vi "tables.vi"() -> ()   [LabVIEW 2018]
panel:
  out "Array":i32[][](array[numeric])
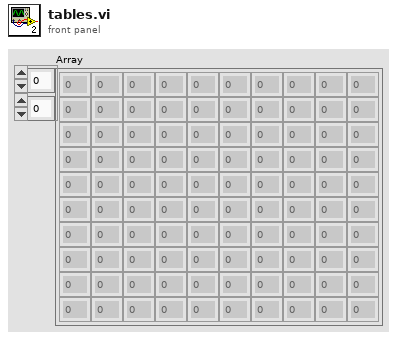
[diagram p1: front panel]
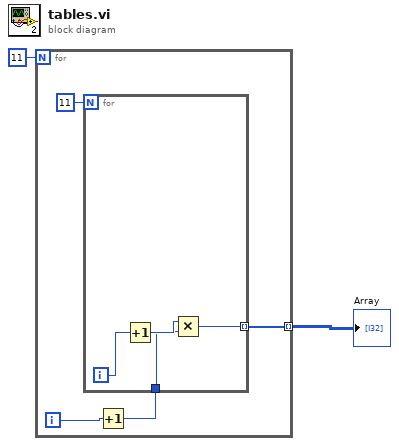
[diagram p0: block diagram]
diagram:
  n1 = for {
    N: 11 -> [_]
    tunnel: [w5] -> w1 mode=indexing
    i -> [w4]
    n2 = Increment(x=w4) -> (x+1=w3:i32)
    n3 = for {
      N: 11 -> [_]
      tunnel: w3 -> [w9]
      tunnel: [w8] -> w5 mode=indexing
      i -> [w7]
      n4 = Increment(x=w7) -> (x+1=w10:i32)
      n5 = Multiply(x=w10, y=w9) -> (x*y=w8:i32)
    }
  }
  "Array" <- w1
